vi "Open Front Panel.vi"(8 "error in (no error)":errorcluster, 11 "Mag Lab Hardware in":refnum<class "Mag Lab Hardware.lvclass">) -> (0 "error out":errorcluster, 3 "Mag Lab Hardware out":refnum<class "Mag Lab Hardware.lvclass">)   [LabVIEW 2015, in "Mag Lab Hardware.lvclass"]
uses:
  Mag Lab Hardware.lvclass
  Mag Lab Properties/Mag Lab Parameters.lvclass
  Mag Lab Measure Base/Mag Lab Measure Base.lvclass
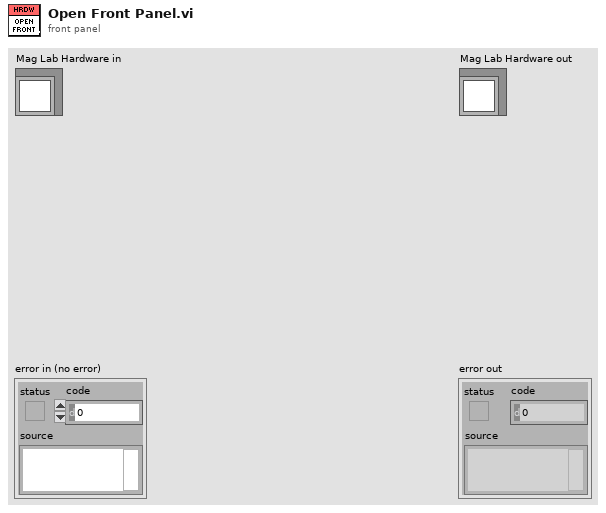
[diagram p1: front panel]
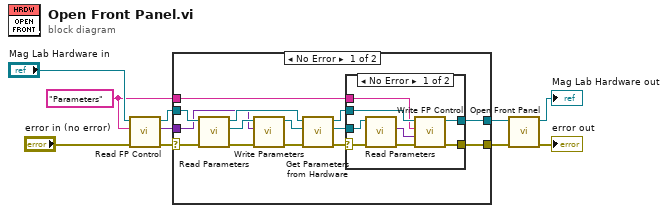
[diagram p0: block diagram]
diagram:
  w4 = "Parameters" ("Control Name")
  n1 = call-dynamic "Read FP Control.vi"("error in (no error)"="error in (no error)", "Control Name"=w4, "Mag Lab Measure Base in"="Mag Lab Hardware in") -> ("error out"=w3:errorcluster, "Control Value"=w1:variant, "Mag Lab Measure Base out"=w2:refnum<class "Mag Lab Hardware.lvclass">)  [unwired: 6 in]
  n2 = case shown="No Error" w3 {
    selector: w3 -> [w17 _]
    tunnel: w2 -> [w18 w34]
    tunnel: w1 -> [w14 _]
    tunnel: [w23 _] -> w6
    tunnel: [w21 w34] -> w5
    tunnel: w4 -> [w19 _]
    frame No Error {
      n3 = call-dynamic "Read Parameters.vi"("error in (no error)"=w17, "Mag Lab Root in"=w18) -> ("error out"=w12:errorcluster, "Mag Lab Parameters.lvclass"=w15:refnum<class "Mag Lab Parameters.lvclass">, "Mag Lab Root out"=w16:refnum<class "Mag Lab Hardware.lvclass">)  [unwired: 7 in]
      n4 = call-dynamic "Write Parameters.vi"("error in (no error)"=w12, "Parameters"=w14, "Mag Lab Parameters in"=w15) -> ("error out"=w11:errorcluster, "Mag Lab Parameters out"=w13:refnum<class "Mag Lab Parameters.lvclass">)  [unwired: 7 in]
      n5 = call-dynamic "Get Parameters from Hardware.vi"("error in (no error)"=w11, "Initial parameters"=w13, "Mag Lab Measure Base in"=w16) -> ("error out"=w24:errorcluster, "Updated parameters"=w20:refnum<class "Mag Lab Parameters.lvclass">, "Mag Lab Measure Base out"=w22:refnum<class "Mag Lab Hardware.lvclass">)  [unwired: 6 in]
      n6 = case shown="No Error" w24 {
        selector: w24 -> [w27 _]
        tunnel: [w32 _] -> w23
        tunnel: w22 -> [w31 w33]
        tunnel: [w30 w33] -> w21
        tunnel: w20 -> [w28 _]
        tunnel: w19 -> [w29 _]
        frame No Error {
          n7 = call-dynamic "Read Parameters.vi"("error in (no error)"=w27, "Mag Lab Parameters in"=w28) -> ("error out"=w26:errorcluster, "Parameters"=w25:variant)  [unwired: 7 in, 1 out]
          n8 = call-dynamic "Write FP Control.vi"("error in (no error)"=w26, "Control Value"=w25, "Control Name"=w29, "Mag Lab Measure Base in"=w31) -> ("error out"=w32:errorcluster, "Mag Lab Measure Base out"=w30:refnum<class "Mag Lab Hardware.lvclass">)  [unwired: 6 in]
        }
        frame Error {
        }
      }
    }
    frame Error {
    }
  }
  n9 = call-parent "Open Front Panel.vi"("error in (no error)"=w6, "Mag Lab Root in"=w5) -> ("error out"=→"error out":errorcluster, "Mag Lab Root out"=→"Mag Lab Hardware out":refnum<class "Mag Lab Hardware.lvclass">)  [unwired: 8 in]
